vi "Generar texto error.vi"(8 "Error In":errorcluster, 10 "Boolean":bool, 11 "Queue in":refnum<queue>) -> (0 "error out":errorcluster, 3 "Mensaje Error":string)   [LabVIEW 2018]
doc: "Este VI toma un Error de la Queue y lo lleva al formato para insertarlo en el Log, el formato es el siguiente:\n\nERROR\nFecha: (Fecha de ocurrencia del error.\nError N°: (Numero del error, segun codigos LabVIEW o Propios del Software ESA).\nDetalle Error: (Texto del error)"
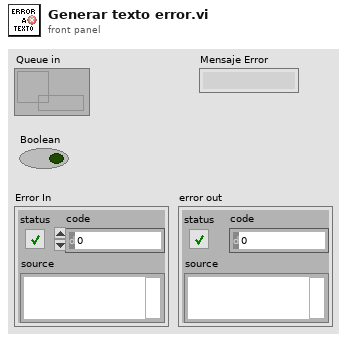
[diagram p1: front panel]
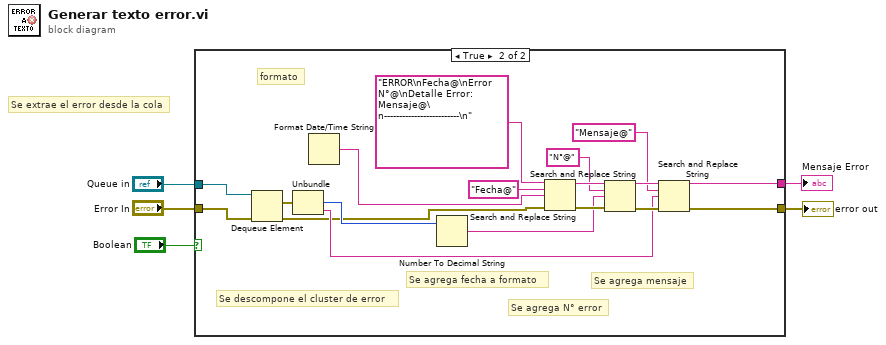
[diagram p0: block diagram]
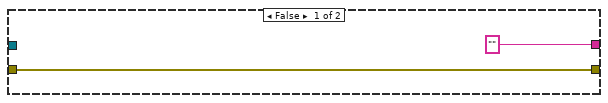
[diagram p2: hidden frame]
diagram:
  # "Se extrae el error desde la cola"
  n1 = case shown="True" "Boolean" {
    tunnel: "Error In" -> [w6 w25]
    tunnel: "Queue in" -> [_ w24]
    tunnel: ["" ("result string") w9] -> w5
    tunnel: [w6 w8] -> w1
    frame False {
    }
    frame True {
      # "Se agrega mensaje"
      # "Se agrega N° error"
      # "Se agrega fecha a formato"
      # "formato"
      # "Se descompone el cluster de error"
      n2 = Dequeue Element(queue=w24, error in (no error)=w25) -> (element=w23:errorcluster, error out=w10:errorcluster)  [unwired: 1 in, 2 out]
      n3 = Unbundle(w23) -> ("code"=w16:i32, "source"=w11:string)  [unwired: 1 out]
      n4 = Format Date/Time String() -> (date/time string=w20:string)  [unwired: 3 in]
      n5 = Number To Decimal String(number=w16) -> (decimal integer string=w15:string)  [unwired: 1 in]
      n6 = Search and Replace String(input string="ERROR\nFecha@\nError N°@\nDetalle Error: Mensaje@\n-------------------------\n", search string="Fecha@", replace string=w20, error in=w10) -> (result string=w18:string, error out=w19:errorcluster)  [unwired: 4 in, 2 out]
      n7 = Search and Replace String(input string=w18, search string="N°@", replace string=w15, error in=w19) -> (result string=w14:string, error out=w13:errorcluster)  [unwired: 4 in, 2 out]
      n8 = Search and Replace String(input string=w14, search string="Mensaje@", replace string=w11, error in=w13) -> (result string=w9:string, error out=w8:errorcluster)  [unwired: 4 in, 2 out]
    }
  }
  "Mensaje Error" <- w5
  "error out" <- w1
